vi "Create_Destination.vi"(8 "error in (no error)":errorcluster, 11 "AB_Destination in":refnum<class "AB_Destination.lvclass">) -> (0 "error out":errorcluster, 2 "directoriesCreated":path[](array[path]), 3 "AB_Destination out":refnum<class "AB_Destination.lvclass">)   [LabVIEW 2020, in "AB_Destination.lvclass"]
uses:
  <vilib>/AppBuilder/AB_Classes/Destination/AB_Destination.lvclass
  <vilib>/AppBuilder/AB_Classes/Destination/AB_Destination.lvclass/AB_Destination.ctl
  <resource>/Framework/Providers/Common/provcom_StringGlobals.vi
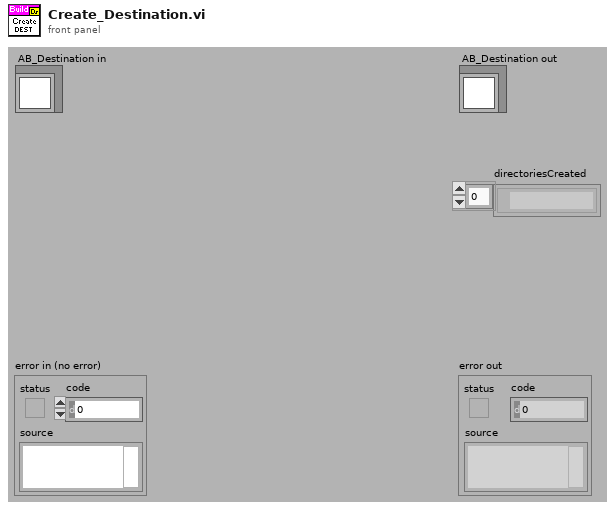
[diagram p1: front panel]
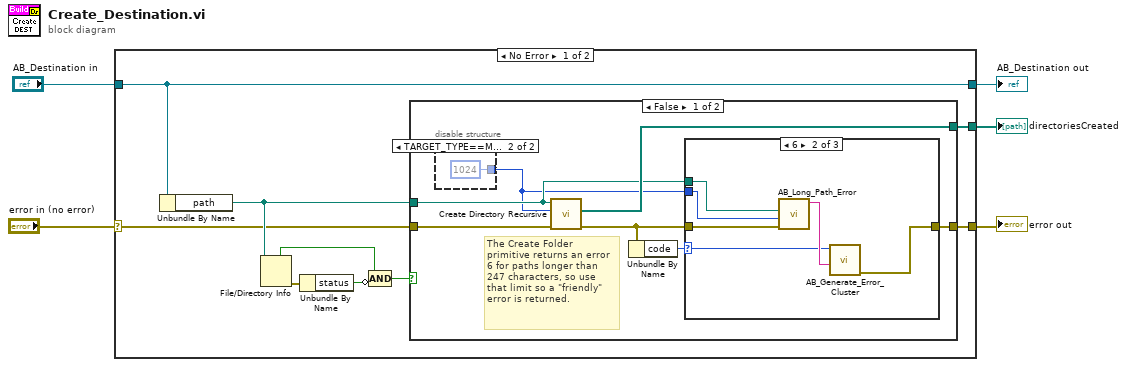
[diagram p0: block diagram]
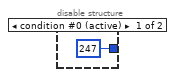
[diagram p2: hidden frame]
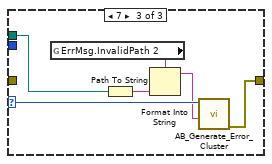
[diagram p4: hidden frame]
diagram:
  n1 = case shown="No Error" "error in (no error)" {
    selector: "error in (no error)" -> [w6 w39]
    tunnel: [w7 w39] -> w4
    tunnel: [w14 w38] -> w2
    tunnel: "AB_Destination in" -> [w14 w38]
    tunnel: [w13 _] -> w1
    frame No Error {
      n2 = Unbundle By Name(w14) -> ("path"=w9:path)
      n3 = File/Directory Info(path=w9) -> (directory=w12:bool, error out=w10:errorcluster)  [unwired: 1 in, 5 out]
      n4 = Unbundle By Name(w10) -> ("status"=w11:bool)
      n5 = Compound Arithmetic op=AND(w12, invert w11) -> (w8:bool)
      n6 = case shown="False" w8 {
        tunnel: [w21 _] -> w13
        tunnel: w9 -> [w16 _]
        tunnel: [w17 w37] -> w7
        tunnel: w6 -> [w20 w37]
        frame False {
          # "The Create Folder primitive returns an error 6 for paths longer than 247 characters, so use that limit so a \"friendly\" error is returned."
          n7 = disable-structure shown="TARGET_TYPE==Mac" {
            disable-tunnel: [247 ("Maximum Allowable Path Length (252)") 1024 ("Maximum Allowable Path Length (252)")] -> w15
            frame condition #0 (active) {
            }
            frame condition #1 {
            }
          }
          n8 = call <vilib>:"Create Directory Recursive.vi"("error in (no error)"=w20, "maximum path length"=w15, "directory"=w16) -> ("error out"=w18:errorcluster, "directories created"=w21:path[])  [unwired: 1 in, 2 out]
          n9 = Unbundle By Name(w18) -> ("code"=w19:i32)
          n10 = case shown="6" w19 {
            selector: w19 -> [_ w27 w35]
            tunnel: w18 -> [w24 w30 _]
            tunnel: [w24 w26 w36] -> w17
            tunnel: w16 -> [_ w29 w32]
            tunnel: w15 -> [_ w25 _]
            frame Default {
            }
            frame 6 {
              n11 = call <vilib>:"AB_Long_Path_Error.vi"("error in (no error)"=w30, "Maximum Allowable Path Length (252)"=w25, "Path"=w29) -> ("error string out"=w28:string)  [unwired: 7 in, 1 out]
              n12 = call <vilib>:"AB_Generate_Error_Cluster.vi"("Additional Message"=w28, "Code"=w27) -> ("error out"=w26:errorcluster)  [unwired: 2 in, 7 out]
            }
            frame 7 {
              n13 = global read "provcom_StringGlobals.vi" "ErrMsg.InvalidPath 2"() -> (w33:string)
              n14 = Path To String(path=w32) -> (string=w34:string)
              n15 = Format Into String(format string=w33, w34) -> (resulting string=w31:string)  [unwired: 2 in, 1 out]
              n16 = call <vilib>:"AB_Generate_Error_Cluster.vi"("Additional Message"=w31, "Code"=w35) -> ("error out"=w36:errorcluster)  [unwired: 2 in, 7 out]
            }
          }
        }
        frame True {
        }
      }
    }
    frame Error {
    }
  }
  "error out" <- w4
  "AB_Destination out" <- w2
  "directoriesCreated" <- w1
